vi "OvertakingDecisor.vi"(0 "Trajectory Network":T1(array[cluster]), 1 "PlatoonArray":i32[](array[numeric]), 3 "Trucks Poses":dbl[][](array[numeric]), 5 "Current State In":i32[](array[numeric]), 7 "Total Platooning Distance":dbl[](array[numeric]), 9 "Set MasterID":i32(ring) items=["None", "Blue Truck", "Black Truck", "Red Truck", "Grey Truck", "DarkGrey Truck"], 11 "CurrentWP":i32[](array[numeric]), 13 "Vref":dbl[](array[numeric])) -> (4 "VrefOut":dbl, 6 "Current WP Out":i32=1, 10 "Set MasterID Out":i32(ring) items=["None", "Blue Truck", "Black Truck", "Red Truck", "Grey Truck", "DarkGrey Truck"], 14 "Current State Out":i32, 15 "Trajectory WP Out":dbl[][](array[numeric]))   [LabVIEW 2013]
uses:
  Global.vi
  <vilib>/imath/engines/lvmath2/RunTimeEngine/ErrorHandling/NIMS_Finalize Error.vi
  <vilib>/imath/engines/lvmath2/RunTimeEngine/VariableToken/NIMS_VariableToken_CondDefined.vi
  <instcachedir>/0/NIMS_VariableToken_CondDefined_9DC5CEC47F8146B087FA2781C705B229.lvgen/NIMS_VariableToken_CondDefined_9DC5CEC47F8146B087FA2781C705B229_004.vi
  <vilib>/imath/engines/lvmath/Functions/Error Handling/MergeErrorsWrapper.vi
  <vilib>/imath/engines/lvmath2/RunTimeEngine/NodeEndStatement/NIMS_NodeEndStatement_Output.vi
  <instcachedir>/0/NIMS_NodeEndStatement_Output_53EC0D466D134D7ABD903AC30B43404B.lvgen/NIMS_NodeEndStatement_Output_53EC0D466D134D7ABD903AC30B43404B_009.vi
  <instcachedir>/0/NIMS_NodeEndStatement_Output_53EC0D466D134D7ABD903AC30B43404B.lvgen/NIMS_NodeEndStatement_Output_53EC0D466D134D7ABD903AC30B43404B_010.vi
  <instcachedir>/0/NIMS_NodeEndStatement_Output_53EC0D466D134D7ABD903AC30B43404B.lvgen/NIMS_NodeEndStatement_Output_53EC0D466D134D7ABD903AC30B43404B_015.vi
  <instcachedir>/0/NIMS_NodeEndStatement_Output_53EC0D466D134D7ABD903AC30B43404B.lvgen/NIMS_NodeEndStatement_Output_53EC0D466D134D7ABD903AC30B43404B_001.vi
  <instcachedir>/0/NIMS_NodeEndStatement_Output_53EC0D466D134D7ABD903AC30B43404B.lvgen/NIMS_NodeEndStatement_Output_53EC0D466D134D7ABD903AC30B43404B_005.vi
  <instcachedir>/0/NIMS_NodeEndStatement_Output_53EC0D466D134D7ABD903AC30B43404B.lvgen/NIMS_NodeEndStatement_Output_53EC0D466D134D7ABD903AC30B43404B_000.vi
  <vilib>/imath/engines/lvmath2/RunTimeEngine/IndexRead/NIMS M($,S).vi
  <instcachedir>/0/NIMS M($,S)_3E5749BBB62E49528D4765A77F1F6D98.lvgen/NIMS M($,S)_3E5749BBB62E49528D4765A77F1F6D98_000.vi
  <vilib>/imath/engines/lvmath2/RunTimeEngine/BuiltInFunctions/deg_to_rad/NIMS_deg_to_rad.vi
  <instcachedir>/0/NIMS_deg_to_rad_4A81D684CE8D4DD79924F5AB74D756E1.lvgen/NIMS_deg_to_rad_4A81D684CE8D4DD79924F5AB74D756E1_002.vi
  <vilib>/imath/engines/lvmath2/RunTimeEngine/IndexReplace/NIMS M($,S)=V.vi
  <instcachedir>/0/NIMS M($,S)=V_D41FDDDB142B47FCA5EF37B60D4970ED.lvgen/NIMS M($,S)=V_D41FDDDB142B47FCA5EF37B60D4970ED_001.vi
  <vilib>/imath/engines/lvmath2/RunTimeEngine/ErrorHandling/NIMS_Create Error From Enums.vi
  <vilib>/imath/engines/lvmath2/RunTimeEngine/IndexRead/NIMS M(S,S).vi
  <instcachedir>/0/NIMS M(S,S)_AC51E74150A542F7991B9634C66F3096.lvgen/NIMS M(S,S)_AC51E74150A542F7991B9634C66F3096_000.vi
  <vilib>/imath/engines/lvmath2/RunTimeEngine/BuiltInFunctions/atan2/NIMS_atan2.vi
  <instcachedir>/0/NIMS_atan2_A91AA4A7D42247EDBE8F76DB99AF04A4.lvgen/NIMS_atan2_A91AA4A7D42247EDBE8F76DB99AF04A4_000.vi
  <vilib>/imath/engines/lvmath2/RunTimeEngine/BuiltInFunctions/rem/NIMS_rem_no checks.vi
  <instcachedir>/0/NIMS_rem_no checks_7935C26835844EFC868069820ED089DA.lvgen/NIMS_rem_no checks_7935C26835844EFC868069820ED089DA_008.vi
  <vilib>/imath/engines/lvmath2/RunTimeEngine/IndexRead/NIMS V(S).vi
  <instcachedir>/0/NIMS V(S)_0488751826AF41519A22953C041130DC.lvgen/NIMS V(S)_0488751826AF41519A22953C041130DC_000.vi
  <vilib>/imathl/engines/lvmath/Functions/Error Handling/Create Error.vi
  <vilib>/imath/engines/lvmath2/RunTimeEngine/ArithmeticOperatorToken/NIMS_ArithmeticOperator_plus.vi
  <instcachedir>/0/NIMS_ArithmeticOperator_plus_8A46DAFC24D445C9B2C97B626139369E.lvgen/NIMS_ArithmeticOperator_plus_8A46DAFC24D445C9B2C97B626139369E_004.vi
  <vilib>/imath/engines/lvmath2/RunTimeEngine/BuiltInFunctions/atan2/NIMS_atan2(A,A).vi
  <instcachedir>/0/NIMS_atan2(A,A)_2936FD7F864E46C682B467FE18724EF9.lvgen/NIMS_atan2(A,A)_2936FD7F864E46C682B467FE18724EF9_004.vi
  <vilib>/imath/engines/lvmath2/RunTimeEngine/ArithmeticOperatorToken/NIMS_ArithmeticOperator_times.vi
  <instcachedir>/0/NIMS_ArithmeticOperator_times_F6527734CE75451889337B8CE94765C6.lvgen/NIMS_ArithmeticOperator_times_F6527734CE75451889337B8CE94765C6_008.vi
  <vilib>/imath/engines/lvmath2/RunTimeEngine/VariableToken/Support/NIMS_Vector Boolean Index to I32 Index.vi
  <vilib>/imath/engines/lvmath2/RunTimeEngine/IndexReplace/NIMS V(V)=S.vi
  <instcachedir>/0/NIMS V(V)=S_43E6004D39A2403BA86EB2871913A93B.lvgen/NIMS V(V)=S_43E6004D39A2403BA86EB2871913A93B_004.vi
  <vilib>/imath/engines/lvmath2/RunTimeEngine/BuiltInFunctions/min/1 input/NIMS_min(CV).vi
  <instcachedir>/0/NIMS_min(CV)_46E60952406B4159AB512BDF500C959F.lvgen/NIMS_min(CV)_46E60952406B4159AB512BDF500C959F_000.vi
  <vilib>/imath/engines/lvmath2/RunTimeEngine/IndexRead/NIMS V(R2).vi
  <instcachedir>/0/NIMS V(R2)_C76619605A0E4E9F8B2FA9389712AC47.lvgen/NIMS V(R2)_C76619605A0E4E9F8B2FA9389712AC47_002.vi
  <vilib>/imath/engines/lvmath2/RunTimeEngine/BuiltInFunctions/findnz/NIMS_[1o]_findnz(GRowV).vi
  <instcachedir>/0/NIMS_[1o]_findnz(GRowV)_A907680C39E74AF18CBD76E991AC1137.lvgen/NIMS_[1o]_findnz(GRowV)_A907680C39E74AF18CBD76E991AC1137_000.vi
  <vilib>/imath/engines/lvmath2/RunTimeEngine/IndexRead/NIMS V(V).vi
  <instcachedir>/0/NIMS V(V)_298D9CB7BFEB42B8BC8D9C3C28AE8C70.lvgen/NIMS V(V)_298D9CB7BFEB42B8BC8D9C3C28AE8C70_000.vi
  <vilib>/imath/engines/lvmath2/RunTimeEngine/BuiltInFunctions/is_empty/NIMS_is_empty(GV).vi
  <instcachedir>/0/NIMS_is_empty(GV)_FC7E7C3D9544432CB6AA2416ADCF6D56.lvgen/NIMS_is_empty(GV)_FC7E7C3D9544432CB6AA2416ADCF6D56_000.vi
  <instcachedir>/0/NIMS V(S)_0488751826AF41519A22953C041130DC.lvgen/NIMS V(S)_0488751826AF41519A22953C041130DC_002.vi
panel:
  out "angle2wp":dbl[](array[numeric])
  out "dist":dbl[](array[numeric])
  out "LeaderDistance":dbl
  out "IsOvertaking":bool
  in  "Platooning Speed  Increment":dbl=1.25
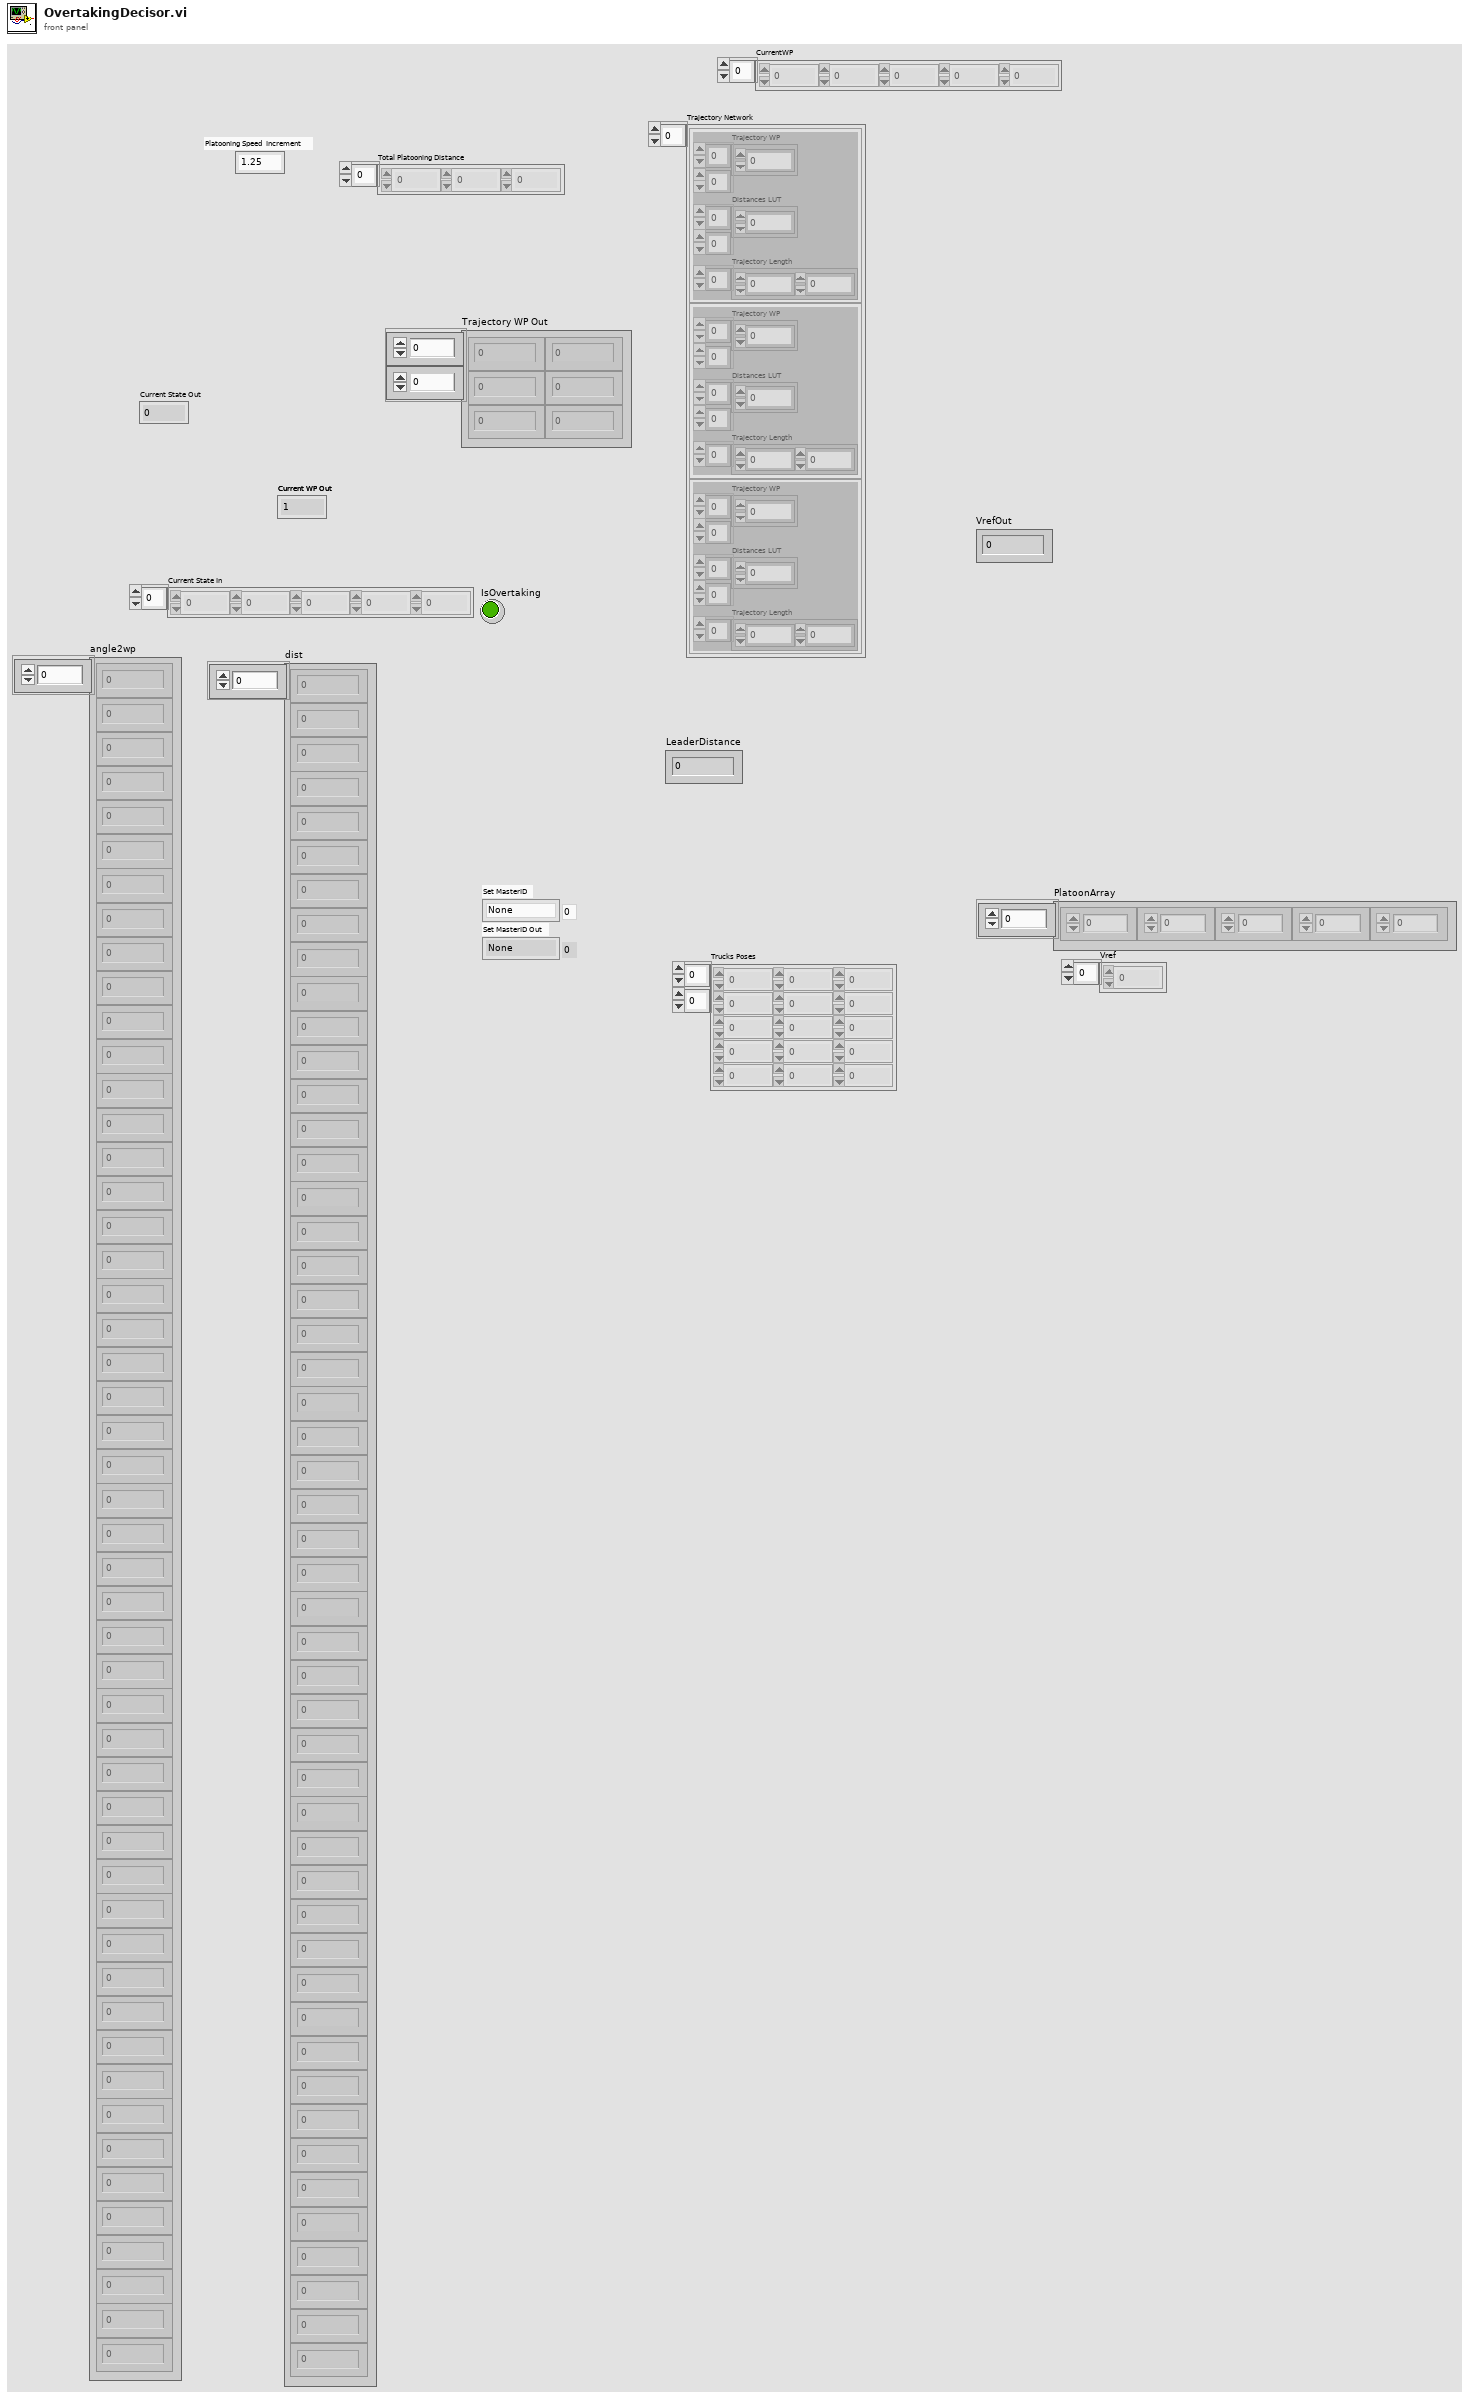
[diagram p1: front panel]
types:
  T1 = cluster{"Trajectory WP":dbl[][], "Distances LUT":dbl[][], "Trajectory Length":i32[]}[]
  T2 = cluster{"Trajectory WP":dbl[][], "Distances LUT":dbl[][], "Trajectory Length":i32[]}
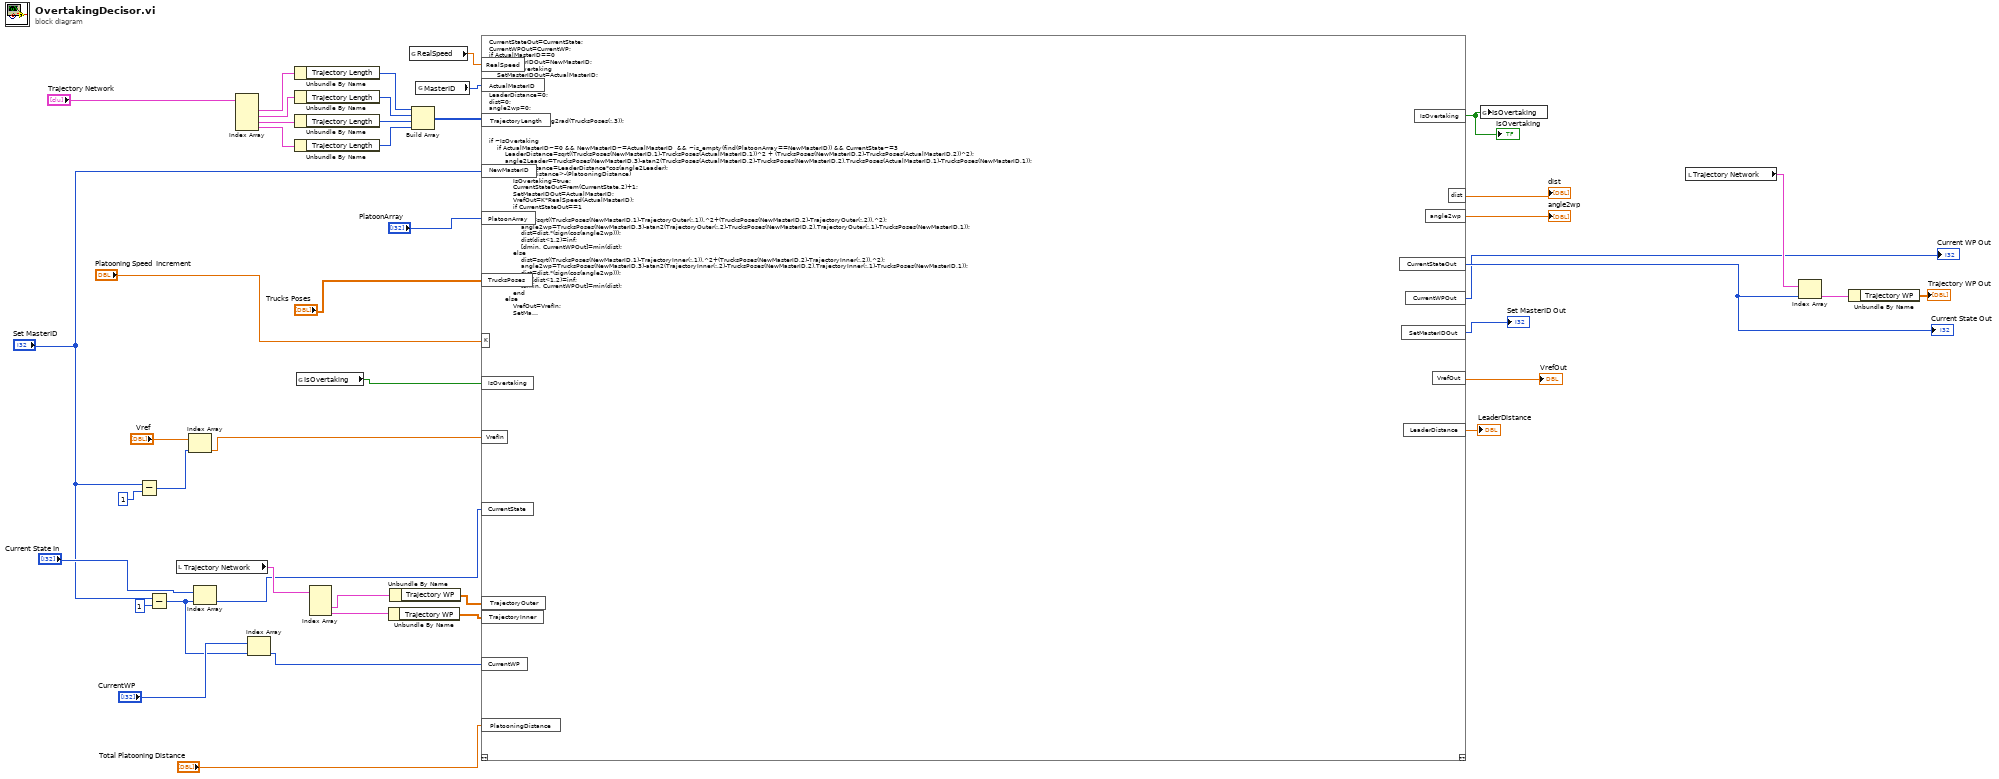
[diagram p0: block diagram]
diagram:
  n1 = Subtract(x="Set MasterID", y=u8 1) -> (x-y=w19:i32)
  n2 = Subtract(x="Set MasterID", y=u8 1) -> (x-y=w9:i32)
  n3 = local read "Trajectory Network"() -> (w32:T1)
  n4 = Index Array(array="Vref", index=w19) -> (element=w18:dbl)
  n5 = Index Array(array="Current State In", index=w9) -> (element=w24:i32)
  n6 = Index Array(array="Trajectory Network") -> (element #1=w40:T2, element #2=w38:T2, element #3=w39:T2, element #4=w37:T2)  [unwired: 4 in]
  n7 = Index Array(array="CurrentWP", index=w9) -> (element=w8:i32)
  n8 = Unbundle By Name(w40) -> ("Trajectory Length"=w44:i32[])
  n9 = Unbundle By Name(w38) -> ("Trajectory Length"=w43:i32[])
  n10 = Unbundle By Name(w39) -> ("Trajectory Length"=w42:i32[])
  n11 = Unbundle By Name(w37) -> ("Trajectory Length"=w36:i32[])
  n12 = global read "Global.vi" "IsOvertaking"() -> (w23:bool)
  n13 = Index Array(array=w32) -> (element #2=w6:T2, element #3=w5:T2)  [unwired: 3 in, 1 out]
  n14 = Unbundle By Name(w5) -> ("Trajectory WP"=w16:dbl[][])
  n15 = Unbundle By Name(w6) -> ("Trajectory WP"=w27:dbl[][])
  n16 = global read "Global.vi" "RealSpeed"() -> (w7:dbl[])
  n17 = Build Array(w44, w43, w42, w36) -> (w26:i32[][])
  n18 = global read "Global.vi" "MasterID"() -> (w25:i32)
  n19 = mathscript code="CurrentStateOut=CurrentState;\nCurrentWPOut=CurrentWP;\nif ActualMasterID==0\n    SetMasterIDOut=NewMasterID;\nelseif ~IsOvertaking\n    SetMasterIDOut=ActualMasterID;\nend\nVrefOut=VrefIn;\nLeaderDistance=0;\ndist=0;\nangle2wp=0;\n\nTrucksPoses(:,3)=deg2rad(TrucksPoses(:,3));\n\n\nif ~IsOvertaking\n    if ActualMasterID~=0 && NewMasterID~=ActualMasterID  && ~is_empty(find(PlatoonArray==NewMasterID)) && CurrentState~=3\n        LeaderDistance=sqrt((TrucksPoses(NewMasterID,1)-TrucksPoses(ActualMasterID,1))^2 + (TrucksPoses(NewMasterID,2)-TrucksPoses(ActualMasterID,2))^2);\n        angle2Leader=TrucksPoses(NewMasterID,3)-atan2(TrucksPoses(ActualMasterID,2)-TrucksPoses(NewMasterID,2),TrucksPoses(ActualMasterID,1)-TrucksPoses(NewMasterID,1));\n        LeaderDistance=LeaderDistance*cos(angle2Leader);\n        if LeaderDistance>-(PlatooningDistance)\n            IsOvertaking=true;\n            CurrentStateOut=rem(CurrentState,2)+1;\n            SetMasterIDOut=ActualMasterID;\n            VrefOut=K*RealSpeed(ActualMasterID);\n            if CurrentStateOut==1\n                \n                dist=sqrt((TrucksPoses(NewMasterID,1)-TrajectoryOuter(:,1)).^2+(TrucksPoses(NewMasterID,2)-TrajectoryOuter(:,2)).^2);\n                angle2wp=TrucksPoses(NewMasterID,3)-atan2(TrajectoryOuter(:,2)-TrucksPoses(NewMasterID,2),TrajectoryOuter(:,1)-TrucksPoses(NewMasterID,1));\n                dist=dist.*(sign(cos(angle2wp)));\n                dist(dist<1.2)=inf;\n                [dmin, CurrentWPOut]=min(dist);\n            else\n                dist=sqrt((TrucksPoses(NewMasterID,1)-TrajectoryInner(:,1)).^2+(TrucksPoses(NewMasterID,2)-TrajectoryInner(:,2)).^2);\n                angle2wp=TrucksPoses(NewMasterID,3)-atan2(TrajectoryInner(:,2)-TrucksPoses(NewMasterID,2),TrajectoryInner(:,1)-TrucksPoses(NewMasterID,1));\n                dist=dist.*(sign(cos(angle2wp)));\n                dist(dist<1.2)=inf;\n                [dmin, CurrentWPOut]=min(dist);\n            end\n        else\n            VrefOut=VrefIn;\n            SetMasterIDOut=NewMasterID;\n            CurrentStateOut=CurrentState;\n            CurrentWPOut=CurrentWP;\n            IsOvertaking=false;\n        end\n    end\n\nelse\n    if ActualMasterID==0\n        ActualMasterID=PlatoonArray(find(PlatoonArray(2:end)~=0,1)+1);\n        if is_empty(ActualMasterID)\n            IsOvertaking=false;\n            CurrentStateOut=rem(CurrentState,2)+1;\n            VrefOut=VrefIn;\n            if CurrentStateOut==1\n                \n                dist=sqrt((TrucksPoses(NewMasterID,1)-TrajectoryOuter(:,1)).^2+(TrucksPoses(NewMasterID,2)-TrajectoryOuter(:,2)).^2);\n                angle2wp=TrucksPoses(NewMasterID,3)-atan2(TrajectoryOuter(:,2)-TrucksPoses(NewMasterID,2),TrajectoryOuter(:,1)-TrucksPoses(NewMasterID,1));\n                dist=dist.*(sign(cos(angle2wp)));\n                dist(dist<1.5)=inf;\n                [dmin, CurrentWPOut]=min(dist);\n            else\n                dist=sqrt((TrucksPoses(NewMasterID,1)-TrajectoryInner(:,1)).^2+(TrucksPoses(NewMasterID,2)-TrajectoryInner(:,2)).^2);\n                angle2wp=TrucksPoses(NewMasterID,3)-atan2(TrajectoryInner(:,2)-TrucksPoses(NewMasterID,2),TrajectoryInner(:,1)-TrucksPoses(NewMasterID,1));\n                dist=dist.*(sign(cos(angle2wp)));\n                dist(dist<1.5)=inf;\n                [dmin, CurrentWPOut]=min(dist);\n            end\n        else\n            ActualMasterID=ActualMasterID(1);\n            LeaderDistance=sqrt((TrucksPoses(NewMasterID,1)-TrucksPoses(ActualMasterID,1))^2 + (TrucksPoses(NewMasterID,2)-TrucksPoses(ActualMasterID,2))^2);\n            angle2Leader=TrucksPoses(NewMasterID,3)-atan2(TrucksPoses(ActualMasterID,2)-TrucksPoses(NewMasterID,2),TrucksPoses(ActualMasterID,1)-TrucksPoses(NewMasterID,1));\n            LeaderDistance=LeaderDistance*cos(angle2Leader);\n            if LeaderDistance<-(PlatooningDistance)\n                IsOvertaking=false;\n                CurrentStateOut=rem(CurrentState,2)+1;\n                VrefOut=K*RealSpeed(ActualMasterID);;\n                if CurrentStateOut==1\n                    \n                    dist=sqrt((TrucksPoses(NewMasterID,1)-TrajectoryOuter(:,1)).^2+(TrucksPoses(NewMasterID,2)-TrajectoryOuter(:,2)).^2);\n                    angle2wp=TrucksPoses(NewMasterID,3)-atan2(TrajectoryOuter(:,2)-TrucksPoses(NewMasterID,2),TrajectoryOuter(:,1)-TrucksPoses(NewMasterID,1));\n                    dist=dist.*(sign(cos(angle2wp)));\n                    dist(dist<1.5)=inf;\n                    [dmin, CurrentWPOut]=min(dist);\n                else\n                    dist=sqrt((TrucksPoses(NewMasterID,1)-TrajectoryInner(:,1)).^2+(TrucksPoses(NewMasterID,2)-TrajectoryInner(:,2)).^2);\n                    angle2wp=TrucksPoses(NewMasterID,3)-atan2(TrajectoryInner(:,2)-TrucksPoses(NewMasterID,2),TrajectoryInner(:,1)-TrucksPoses(NewMasterID,1));\n                    dist=dist.*(sign(cos(angle2wp)));\n                    dist(dist<1.5)=inf;\n                    [dmin, CurrentWPOut]=min(dist);\n                end\n                SetMasterIDOut=NewMasterID;\n            else\n                SetMasterIDOut=ActualMasterID;\n            end\n        end\n    else\n        LeaderDistance=sqrt((TrucksPoses(NewMasterID,1)-TrucksPoses(ActualMasterID,1))^2 + (TrucksPoses(NewMasterID,2)-TrucksPoses(ActualMasterID,2))^2);\n        angle2Leader=TrucksPoses(NewMasterID,3)-atan2(TrucksPoses(ActualMasterID,2)-TrucksPoses(NewMasterID,2),TrucksPoses(ActualMasterID,1)-TrucksPoses(NewMasterID,1));\n        LeaderDistance=LeaderDistance*cos(angle2Leader);\n        if LeaderDistance<-(PlatooningDistance)\n            IsOvertaking=false;\n            CurrentStateOut=rem(CurrentState,2)+1;\n            VrefOut=K*RealSpeed(ActualMasterID);;\n            if CurrentStateOut==1\n                \n                dist=sqrt((TrucksPoses(NewMasterID,1)-TrajectoryOuter(:,1)).^2+(TrucksPoses(NewMasterID,2)-TrajectoryOuter(:,2)).^2);\n                angle2wp=TrucksPoses(NewMasterID,3)-atan2(TrajectoryOuter(:,2)-TrucksPoses(NewMasterID,2),TrajectoryOuter(:,1)-TrucksPoses(NewMasterID,1));\n                dist=dist.*(sign(cos(angle2wp)));\n                dist(dist<1.5)=inf;\n                [dmin, CurrentWPOut]=min(dist);\n            else\n                dist=sqrt((TrucksPoses(NewMasterID,1)-TrajectoryInner(:,1)).^2+(TrucksPoses(NewMasterID,2)-TrajectoryInner(:,2)).^2);\n                angle2wp=TrucksPoses(NewMasterID,3)-atan2(TrajectoryInner(:,2)-TrucksPoses(NewMasterID,2),TrajectoryInner(:,1)-TrucksPoses(NewMasterID,1));\n                dist=dist.*(sign(cos(angle2wp)));\n                dist(dist<1.5)=inf;\n                [dmin, CurrentWPOut]=min(dist);\n            end\n            SetMasterIDOut=NewMasterID;\n        else\n            SetMasterIDOut=ActualMasterID;\n        end\n    end\nend"("ActualMasterID"=w25, "NewMasterID"="Set MasterID", "PlatoonArray"="PlatoonArray", "TrucksPoses"="Trucks Poses", "TrajectoryOuter"=w27, "TrajectoryLength"=w26, "CurrentState"=w24, "IsOvertaking"=w23, "VrefIn"=w18, "K"="Platooning Speed  Increment", "TrajectoryInner"=w16, "CurrentWP"=w8, "RealSpeed"=w7, "PlatooningDistance"="Total Platooning Distance") -> ("IsOvertaking"=w15:bool, "SetMasterIDOut"=→"Set MasterID Out":i32, "VrefOut"=→"VrefOut":dbl, "CurrentStateOut"=w14:i32, "CurrentWPOut"=→"Current WP Out":i32, "LeaderDistance"=→"LeaderDistance":cdb, "dist"=→"dist":cdb[], "angle2wp"=→"angle2wp":dbl[])  [unwired: 1 in, 1 out]
  "Current State Out" <- w14
  "IsOvertaking" <- w15
  n20 = global write "Global.vi" "IsOvertaking"(w15) -> ()
  n21 = local read "Trajectory Network"() -> (w33:T1)
  n22 = Index Array(array=w33, index=w14) -> (element=w35:T2)
  n23 = Unbundle By Name(w35) -> ("Trajectory WP"=→"Trajectory WP Out":dbl[][])
